vi "RFmxSpecAn CHP (Analysis Only).vi"() -> ()   [LabVIEW 2017]
doc: "This example illustrates how to use NI-RFmx in hardware agnostic mode to perform measurements on user provided IQ or Spectrum waveform. The example uses NI-RFSA driver API to acquire waveform from NI RF Signal Analyzer and perform an ACP measurement. The NI-RFSA acquisition settings are read from NI-RFmx session after Commit VI call. The NI-RFmx session is opened with Option String set as \"AnalysisOnly=1\"."
uses:
  <instrlib>/niRFSA/niRFSA.llb/niRFSA Ref Clock Sources.ctl
  <instrlib>/niRFSA/niRFSA.llb/niRFSA Exported Signal Destinations.ctl
  <instrlib>/niRFSA/niRFSA.llb/niRFSA Trigger Terminals.ctl
  <vilib>/Utility/error.llb/DialogType.ctl
  <instrlib>/niRFSA/niRFSA.llb/niRFSA Acquisition Types.ctl
  <instrlib>/niRFSA/niRFSA.llb/niRFSA Signal Names.ctl
  <vilib>/RFmx/SpecAn/mx/RFmxSpecAn.llb/RFmxSpecAn Select Measurement (Single).vi
  <instrlib>/niRFSA/niRFSA.llb/niRFSA Configure Digital Edge Advance Trigger.vi
  <instrlib>/niRFSA/niRFSA.llb/niRFSA Fetch IQ (1D Complex WDT NRec 1Chan).vi
  <vilib>/RFmx/SpecAn/mx/RFmxSpecAn.llb/RFmxSpecAn Analyze (IQ).vi
  <vilib>/RFmx/SpecAn/mx/RFmxSpecAn.llb/RFmxSpecAn CHP Fetch Measurement.vi
  <vilib>/RFmx/SpecAn/mx/RFmxSpecAn.llb/RFmxSpecAn CHP Fetch Spectrum.vi
  <vilib>/measure/maspectr.llb/FFT Power Spectrum and PSD for 1 Chan (CDB).vi
  <vilib>/measure/NI_MAPro.lvlib
  <instrlib>/niRFSA/niRFSA.llb/niRFSA Configure Digital Edge Start Trigger.vi
  <vilib>/measure/maspectr.llb/FFT Power Spectrum and PSD for 1 Chan.vi
  <resource>/objmgr/RFmxInstr.rc
panel:
  out "Recommended Meas BW (Hz)":dbl
  out "Recommended Min Sample Rate (Hz)":dbl format="%#_6p"
  out "Recommended Acquisition Time (s)":dbl
  out "Waveform Graph 2":cluster{"x0":dbl, "dx":dbl, "y":sgl[]}(graph)
  out "Waveform Graph":cluster{"f0":dbl, "df":dbl, "magnitude":dbl[]}(graph)
  out "Absolute Power (dBm)":dbl format="%.2f"
  out "Signal Path:IF Filter Bandwidth":dbl format="%#_6p"
  out "Signal Path:LO Frequency":dbl format="%#_6p"
  in  "number of records":i64=5
  in  "source":T1="PXI_Trig0"
  in  "output terminal":T2="PXI_Trig1"
  in  "Carrier Frequency (Hz)":dbl=4000000000.0 format="%#_6p"
  in  "Clock Source":T3="OnboardClock"
  in  "Resource Name 2":refnum<k15>="RFSA" caption="Resource Name"
  in  "Resolution Bandwidth (Hz)":dbl=10000.0 format="%#_6p"
  in  "Reference Level (dBm) 2":dbl caption="Reference Level (dBm)" format="%.2f"
  in  "Span (Hz)":dbl=765000000.0 format="%.3p"
  in  "Integration Bandwidth (Hz)":dbl=1000000.0 format="%.3p"
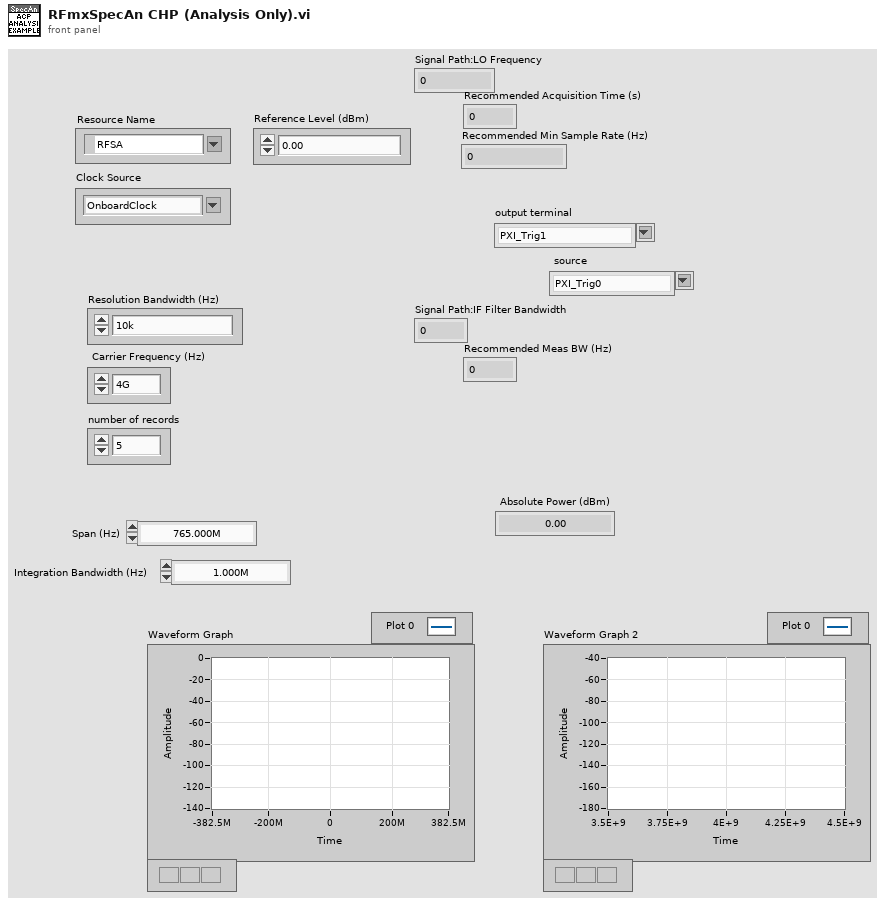
[diagram p1: front panel]
types:
  T1 = typedef "niRFSA Trigger Terminals.ctl" = string
  T2 = typedef "niRFSA Exported Signal Destinations.ctl" = string
  T3 = typedef "niRFSA Ref Clock Sources.ctl" = string
  T4 = typedef "niRFSA Signal Names.ctl" = i32
  T5 = typedef "niRFSA Acquisition Types.ctl" = i32
  T6 = typedef "DialogType.ctl" = u16
  T7 = enum16{"ACP", "CCDF", "CHP", "FCnt", "Harmonics", "OBW", "SEM", "Spectrum", "Spur", "TXP", "AMPM", "DPD", "IQ", "IM", "NF", "PhaseNoise"}
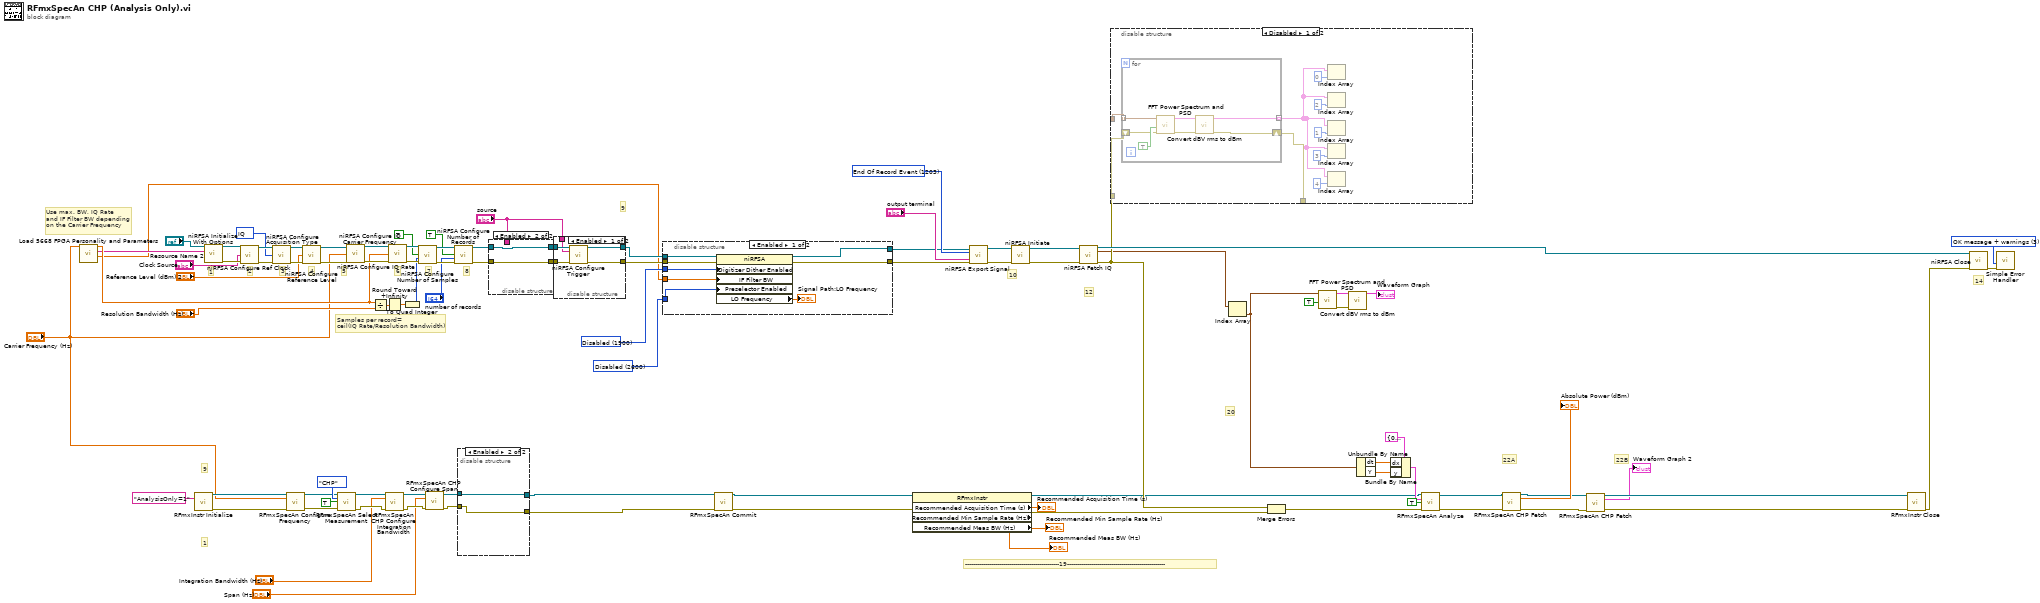
[diagram p0: block diagram]
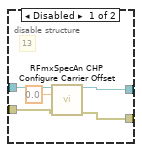
[diagram p2: hidden frame]
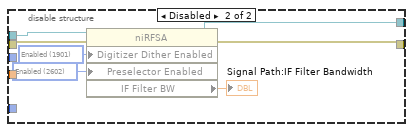
[diagram p4: hidden frame]
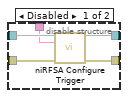
[diagram p6: hidden frame]
diagram:
  w40 = 2600 items=["Disabled"=2600, "Enabled when in Signal Path"=2601, "Enabled"=2602] ("Signal Path:Advanced:Downconverter Preselector Enabled")
  w41 = 1900 items=["Disabled"=1900, "Enabled"=1901] ("Signal Path:Digitizer Dither Enabled")
  w60 = T4 1203 items=["Start Trigger"=1100, "Ref Trigger"=702, "Advance Trigger"=1102, "Ready For Start Event"=1200, "Ready For Ref Event"=1201, "Ready For Advance Event"=1202, "End Of Record Event"=1203, "Done Event"=1204, "Reference Clock"=1205, "User"=1206] ("signal")
  w63 = T5 100 items=["IQ"=100, "Spectrum"=101] ("acquisition type")
  w69 = T6 3 items=["no dialog", "OK message", "continue or stop message", "OK message + warnings", "continue/stop + warnings"] ("type of dialog (OK msg:1)")
  # "22B"
  # "22A"
  # "Use max. BW, IQ Rate \nand IF Filter BW depending \non the Carrier Frequency"
  # "Samples per record= \nceil(IQ Rate/Resolution Bandwidth)"
  # "9"
  # "12"
  # "10"
  # "8"
  # "14"
  # "7"
  # "6"
  # "5"
  # "4"
  # "3"
  # "2"
  # "1"
  # "20"
  # "-----------------------------------------------19-------------------------------------------------"
  # "9"
  # "1"
  n1 = call "Load 5668 FPGA Personality and Parameters.vi"("Start Carrier Frequency in"="Carrier Frequency (Hz)") -> ("Signal Path:IF Filter Bandwidth"=w36:dbl, "option string"=w37:string, "IQ rate (S/s)"=w38:dbl)  [unwired: 8 in]
  n2 = call <vilib>:"RFmxInstr Initialize.vi"("Option String"="AnalysisOnly=1") -> ("Instrument Handle Out"=w93:refnum<k21>, "error out"=w92:errorcluster)  [unwired: 12 in, 1 out]
  n3 = call <instrlib>:"niRFSA Initialize With Options.vi"("resource name"="Resource Name 2", "option string"=w37) -> ("instrument handle out"=w80:refnum<k15>, "error out"=w79:errorcluster)  [unwired: 12 in]
  n4 = call <instrlib>:"niRFSA Configure Ref Clock.vi"("instrument handle"=w80, "clock source"="Clock Source", "error in"=w79) -> ("instrument handle out"=w75:refnum<k15>, "error out"=w76:errorcluster)  [unwired: 11 in]
  n5 = call <instrlib>:"niRFSA Configure Acquisition Type.vi"("instrument handle"=w75, "acquisition type"=w63, "error in"=w76) -> ("instrument handle out"=w78:refnum<k15>, "error out"=w77:errorcluster)  [unwired: 11 in]
  n6 = call <vilib>:"RFmxSpecAn Configure Frequency.vi"("Instrument Handle In"=w93, "Center Frequency (Hz)"="Carrier Frequency (Hz)", "error in (no error)"=w92) -> ("Instrument Handle Out"=w88:refnum<k21>, "error out"=w87:errorcluster)  [unwired: 11 in]
  n7 = call <instrlib>:"niRFSA Configure Reference Level.vi"("instrument handle"=w78, "reference level (dBm)"="Reference Level (dBm) 2", "error in"=w77) -> ("instrument handle out"=w57:refnum<k15>, "error out"=w55:errorcluster)  [unwired: 11 in]
  n8 = call-poly <vilib>:"RFmxSpecAn Select Measurement.vi"("Instrument Handle In"=w88, "Measurement"=T7."CHP", "Enable All Traces"=TRUE, "error in (no error)"=w87) -> ("Instrument Handle Out"=w86:refnum<k21>, "error out"=w85:errorcluster)  [unwired: 10 in]
  n9 = call <instrlib>:"niRFSA Configure IQ Carrier Frequency.vi"("instrument handle"=w57, "carrier frequency"="Carrier Frequency (Hz)", "error in"=w55) -> ("instrument handle out"=w56:refnum<k15>, "error out"=w54:errorcluster)  [unwired: 11 in]
  n10 = Divide(x=w38, y="Resolution Bandwidth (Hz)") -> (x/y=w47:dbl)
  n11 = call <vilib>:"RFmxSpecAn CHP Configure Integration Bandwidth.vi"("Instrument Handle In"=w86, "Integration Bandwidth (Hz)"="Integration Bandwidth (Hz)", "error in (no error)"=w85) -> ("Instrument Handle Out"=w83:refnum<k21>, "error out"=w82:errorcluster)  [unwired: 11 in]
  n12 = Round Toward +Infinity(x=w47) -> (ceil(x): smallest int >= x=w46:dbl)
  n13 = call <instrlib>:"niRFSA Configure IQ Rate.vi"("instrument handle"=w56, "IQ rate (S/s)"=w38, "error in"=w54) -> ("instrument handle out"=w73:refnum<k15>, "error out"=w74:errorcluster)  [unwired: 11 in]
  n14 = To Quad Integer(1:w46) -> (0:w45:i64)
  n15 = call <instrlib>:"niRFSA Configure Number of Samples.vi"("instrument handle"=w73, "number of samples is finite"=TRUE, "samples per record"=w45, "error in"=w74) -> ("instrument handle out"=w68:refnum<k15>, "error out"=w67:errorcluster)  [unwired: 10 in]
  n16 = call <vilib>:"RFmxSpecAn CHP Configure Span.vi"("Instrument Handle In"=w83, "Span (Hz)"="Span (Hz)", "error in (no error)"=w82) -> ("Instrument Handle Out"=w31:refnum<k21>, "error out"=w32:errorcluster)  [unwired: 11 in]
  n17 = call <instrlib>:"niRFSA Configure Number of Records.vi"("instrument handle"=w68, "number of records is finite"=TRUE, "number of records"="number of records", "error in"=w67) -> ("instrument handle out"=w51:refnum<k15>, "error out"=w61:errorcluster)  [unwired: 10 in]
  n18 = disable-structure shown="Enabled" {
    disable-tunnel: w32 -> [w100 w101]
    disable-tunnel: [w99 w101] -> w8
    disable-tunnel: w31 -> [w98 w102]
    disable-tunnel: [w97 w102] -> w2
    frame Disabled {
      # "13"
      n19 = call <vilib>:"RFmxSpecAn CHP Configure Carrier Offset.vi"("Instrument Handle In"=w98, "Carrier Frequency (Hz)"=0.0, "error in (no error)"=w100) -> ("Instrument Handle Out"=w97:refnum<k21>, "error out"=w99:errorcluster)  [unwired: 11 in]
    }
    frame Enabled {
    }
  }
  n20 = disable-structure shown="Enabled" {
    disable-tunnel: w61 -> [w107 w108]
    disable-tunnel: [w106 w108] -> w52
    disable-tunnel: w51 -> [w105 w109]
    disable-tunnel: [w104 w109] -> w50
    disable-tunnel: "source" -> [w103 _]
    frame Disabled {
      n21 = call-poly <instrlib>:"niRFSA Configure Trigger.vi"("instrument handle"=w105, "source"=w103, "error in"=w107) -> ("instrument handle out"=w104:refnum<k15>, "error out"=w106:errorcluster)  [unwired: 11 in]
    }
    frame Enabled {
    }
  }
  n22 = disable-structure shown="Enabled" {
    disable-tunnel: [w114 w115] -> w53
    disable-tunnel: [w113 w116] -> w43
    disable-tunnel: w52 -> [w112 w115]
    disable-tunnel: w50 -> [w111 w116]
    disable-tunnel: "source" -> [w110 _]
    frame Enabled {
      n23 = call-poly <instrlib>:"niRFSA Configure Trigger.vi"("instrument handle"=w111, "source"=w110, "error in"=w112) -> ("instrument handle out"=w113:refnum<k15>, "error out"=w114:errorcluster)  [unwired: 11 in]
    }
    frame Disabled {
    }
  }
  n24 = disable-structure shown="Enabled" {
    disable-tunnel: w53 -> [w124 w129]
    disable-tunnel: [w123 w128] -> w44
    disable-tunnel: w43 -> [w122 w131]
    disable-tunnel: [w121 w130] -> w42
    disable-tunnel: w41 -> [w120 _]
    disable-tunnel: w40 -> [w119 _]
    disable-tunnel: w36 -> [w118 _]
    frame Enabled {
      n25 = property class="niRFSA"(reference=w122, error in=w124, "Digitizer Dither Enabled"=w120, "IF Filter BW"=w118, "Preselector Enabled"=w119) -> (reference out=w121:refnum<k15>, error out=w123:errorcluster, "LO Frequency"=→"Signal Path:LO Frequency":dbl)
    }
    frame Disabled {
      w126 = 2602 items=["Disabled"=2600, "Enabled when in Signal Path"=2601, "Enabled"=2602] ("Signal Path:Advanced:Downconverter Preselector Enabled")
      w127 = 1901 items=["Disabled"=1900, "Enabled"=1901] ("Signal Path:Digitizer Dither Enabled")
      n26 = property class="niRFSA"(reference=w131, error in=w129, "Digitizer Dither Enabled"=w127, "Preselector Enabled"=w126) -> (reference out=w130:refnum<k15>, error out=w128:errorcluster, "IF Filter BW"=→"Signal Path:IF Filter Bandwidth":dbl)
    }
  }
  n27 = call <vilib>:"RFmxSpecAn Commit.vi"("Instrument Handle In"=w2, "error in (no error)"=w8) -> ("Instrument Handle Out"=w1:refnum<k21>, "error out"=w3:errorcluster)  [unwired: 12 in]
  n28 = property class="RFmxInstr"(reference=w1, error in=w3) -> (reference out=w9:refnum<k21>, error out=w7:errorcluster, "Recommended Acquisition Time (s)"=→"Recommended Acquisition Time (s)":dbl, "Recommended Min Sample Rate (Hz)"=→"Recommended Min Sample Rate (Hz)":dbl, "Recommended Meas BW (Hz)"=→"Recommended Meas BW (Hz)":dbl)
  n29 = call <instrlib>:"niRFSA Export Signal.vi"("instrument handle"=w42, "signal"=w60, "output terminal"="output terminal", "error in"=w44) -> ("instrument handle out"=w58:refnum<k15>, "error out"=w30:errorcluster)  [unwired: 10 in]
  n30 = call <instrlib>:"niRFSA Initiate.vi"("instrument handle"=w58, "error in"=w30) -> ("instrument handle out"=w34:refnum<k15>, "error out"=w35:errorcluster)  [unwired: 12 in]
  n31 = call-poly <instrlib>:"niRFSA Fetch IQ.vi"("instrument handle"=w34, "error in"=w35) -> ("instrument handle out"=w65:refnum<k15>, "data"=w23:waveform(cdb)[], "error out"=w29:errorcluster)  [unwired: 11 in]
  n32 = disable-structure shown="Disabled" {
    disable-tunnel: [w140 _] -> _
    disable-tunnel: w29 -> [w133 _]
    disable-tunnel: _ -> [w132 _]
    frame Disabled {
      n33 = for {
        tunnel: w132 -> [w151] mode=indexing
        tunnel: [w146] -> w139 mode=indexing
        shift-right: [w147] -> w140
        shift-left: w133 -> [w150]
        n34 = call-poly <vilib>:"FFT Power Spectrum and PSD.vi"("error in (no error)"=w150, "dB On (F)"=TRUE, "time signal"=w151) -> ("error out"=w148:errorcluster, "Power Spectrum / PSD"=w149:cluster{"f0":dbl, "df":dbl, "magnitude":dbl[]})  [unwired: 5 in, 2 out]
        n35 = call "Convert dBV rms to dBm.vi"("error in (no error)"=w148, "Power Spectrum / PSD (dBV rms)"=w149) -> ("error out"=w147:errorcluster, "Power Spectrum / PSD (dBm)"=w146:cluster{"f0":dbl, "df":dbl, "magnitude":dbl[]})  [unwired: 8 in]
      }
      n36 = Index Array(array=w139, index=3) -> (element=w137:cluster{"f0":dbl, "df":dbl, "magnitude":dbl[]})
      n37 = Index Array(array=w139, index=4) -> (element=w138:cluster{"f0":dbl, "df":dbl, "magnitude":dbl[]})
      n38 = Index Array(array=w139, index=0) -> (element=w134:cluster{"f0":dbl, "df":dbl, "magnitude":dbl[]})
      n39 = Index Array(array=w139, index=2) -> (element=w136:cluster{"f0":dbl, "df":dbl, "magnitude":dbl[]})
      n40 = Index Array(array=w139, index=1) -> (element=w135:cluster{"f0":dbl, "df":dbl, "magnitude":dbl[]})
    }
    frame Enabled {
    }
  }
  n41 = Index Array(array=w23) -> (element=w17:waveform(cdb))  [unwired: 1 in]
  n42 = Merge Errors(w29, w7) -> (w90:errorcluster)
  n43 = call-poly <vilib>:"FFT Power Spectrum and PSD.vi"("dB On (F)"=TRUE, "time signal"=w17) -> ("error out"=w19:errorcluster, "Power Spectrum / PSD"=w18:cluster{"f0":dbl, "df":dbl, "magnitude":dbl[]})  [unwired: 6 in, 2 out]
  n44 = call "Convert dBV rms to dBm.vi"("error in (no error)"=w19, "Power Spectrum / PSD (dBV rms)"=w18) -> ("Power Spectrum / PSD (dBm)"=→"Waveform Graph":cluster{"f0":dbl, "df":dbl, "magnitude":dbl[]})  [unwired: 8 in, 1 out]
  n45 = Unbundle By Name(w17) -> ("dt"=w22:dbl, "Y"=w21:cdb[])
  n46 = Bundle By Name(cluster=cluster{"x0":dbl, "dx":dbl, "y":csg[]} {"x0"=0.0, "dx"=0.0, "y"=[]} ("IQ"), "dx"=w22, "y"=w21) -> (w25:cluster{"x0":dbl, "dx":dbl, "y":csg[]})
  n47 = call-poly <vilib>:"RFmxSpecAn Analyze.vi"("Instrument Handle In"=w9, "IQ"=w25, "Reset?"=TRUE, "error in (no error)"=w90) -> ("Instrument Handle Out"=w28:refnum<k21>, "error out"=w27:errorcluster)  [unwired: 8 in, 2 out]
  n48 = call-poly <vilib>:"RFmxSpecAn CHP Fetch.vi"("Instrument Handle In"=w28, "error in (no error)"=w27) -> ("Instrument Handle Out"=w14:refnum<k21>, "Absolute Power (dBm)"=→"Absolute Power (dBm)":dbl, "error out"=w12:errorcluster)  [unwired: 8 in, 3 out]
  n49 = call-poly <vilib>:"RFmxSpecAn CHP Fetch.vi"("Instrument Handle In"=w14, "error in (no error)"=w12) -> ("Instrument Handle Out"=w13:refnum<k21>, "Spectrum (dBm)"=→"Waveform Graph 2":cluster{"x0":dbl, "dx":dbl, "y":sgl[]}, "error out"=w11:errorcluster)  [unwired: 11 in]
  n50 = call <vilib>:"RFmxInstr Close.vi"("Instrument Handle In"=w13, "error in (no error)"=w11) -> ("error out"=w89:errorcluster)  [unwired: 13 in]
  n51 = call <instrlib>:"niRFSA Close.vi"("instrument handle"=w65, "error in"=w89) -> ("error out"=w72:errorcluster)  [unwired: 13 in]
  n52 = call <vilib>:"Simple Error Handler.vi"("type of dialog (OK msg:1)"=w69, "error in (no error)"=w72) -> ()  [unwired: 3 in, 5 out]
